vi "DB2.NewSettingsConfig.vi"(8 "error in":errorcluster, 10 "New Settings Config":T1, 11 "DB2.lvclass":refnum<class "DB2.lvclass">) -> (0 "error out":errorcluster, 3 "DB2.lvclass":refnum<class "DB2.lvclass">)   [LabVIEW 2022 SP3, in "DB2.lvclass"]
uses:
  DB2.lvclass
  Typedefs/PublicEvents--DB2.NewSettingsConfig.ctl
  DB2.lvclass/DB2.ctl
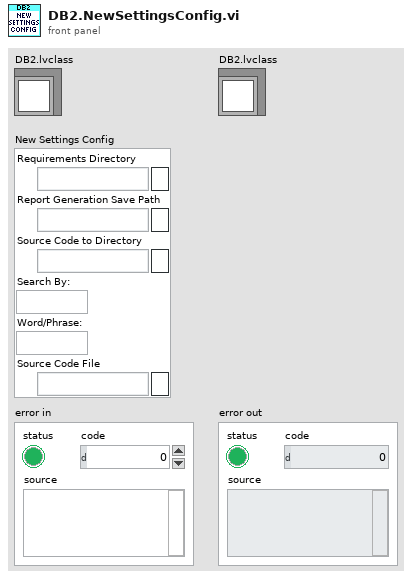
[diagram p1: front panel]
types:
  T1 = typedef "DB2.lvclass/PublicEvents--DB2.NewSettingsConfig.ctl" = cluster{"Requirements Directory":path, "Report Generation Save Path":path, "Source Code to Directory":path, "Search By:":string, "Word/Phrase:":string, "Source Code File":path}
  T2 = typedef "DB2.lvclass/PrivateData--Ref.ctl" = refnum<data-value>
  T3 = typedef "DB2.lvclass/PublicEvents--Cluster.ctl" = cluster{"UI State":refnum<user-event>, "NewSettingsConfig":refnum<user-event>}
  T4 = typedef "DB2.lvclass/DB2 State--enum.ctl" = enum16{"unknown", "Opened", "Embedded", "Closed"}
  T5 = cluster{"Public Events":T3, "Subpanel Ref":refnum<vi>, "UI State":T4}
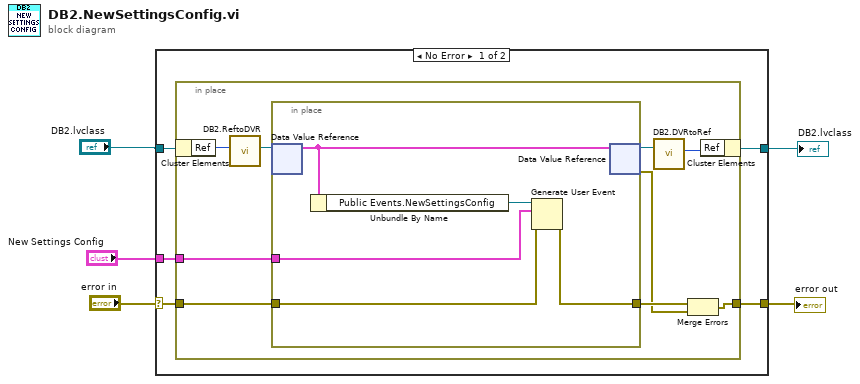
[diagram p0: block diagram]
diagram:
  n1 = case shown="No Error" "error in" {
    selector: "error in" -> [w8 w26]
    tunnel: [w7 w26] -> w2
    tunnel: [w9 w25] -> w4
    tunnel: "DB2.lvclass" -> [w10 w25]
    tunnel: "New Settings Config" -> [w6 _]
    frame No Error {
      n2 = in-place {
        in-place-border: w8 -> [w19]
        in-place-border: [w16] -> w7
        in-place-border: w6 -> [w11]
        n3 = in-place-cluster #1(w10) -> ("Ref"=w15:u32)
        n4 = call "DB2.ReftoDVR.vi"("Ref"=w15) -> ("Ref"=w14:T2)  [unwired: 10 in]
        n5 = in-place {
          in-place-border: w19 -> [w22]
          in-place-border: [w21] -> w18
          in-place-border: w11 -> [w20]
          n6 = in-place-dvr #2(w14) -> (w24:T5)  [unwired: 1 out]
          n7 = Unbundle By Name(w24) -> ("Public Events.NewSettingsConfig"=w23:refnum<user-event>)
          n8 = Generate User Event(user event=w23, event data cluster=w20, error in=w22) -> (error out=w21:errorcluster)  [unwired: 1 in, 1 out]
          n9 = in-place-dvr #2(w24) -> (w13:T2, w17:errorcluster)
        }
        n10 = call "DB2.DVRtoRef.vi"("Ref"=w13) -> ("Ref"=w12:u32)  [unwired: 10 in]
        n11 = Merge Errors(w18, w17) -> (w16:errorcluster)
        n12 = in-place-cluster #1("Ref"=w12) -> (w9:refnum<class "DB2.lvclass">)
      }
    }
    frame Error {
    }
  }
  "DB2.lvclass" <- w4
  "error out" <- w2
